vi "main.vi"(8 "error in (no error)":errorcluster) -> (0 "error out":errorcluster)   [LabVIEW 2018]
doc: "Main VI."
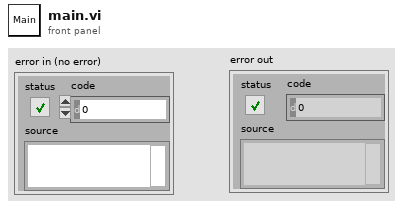
[diagram p1: front panel]
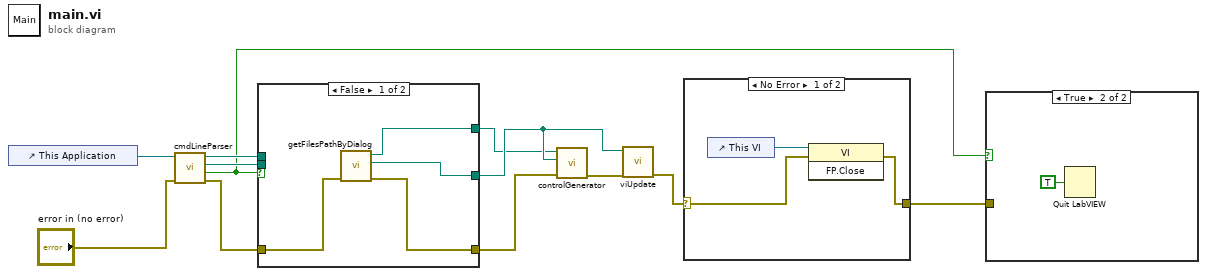
[diagram p0: block diagram]
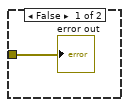
[diagram p2: hidden frame]
diagram:
  n1 = control-ref of="This Application"() -> (w3:refnum<vi>)
  n2 = call "cmdLineParser.vi"("error in (no error)"="error in (no error)", "reference"=w3) -> ("error out"=w9:errorcluster, "filesExist"=w5:bool, "pathLvlibDir"=w7:path, "pathIdl"=w8:path)  [unwired: 6 in]
  n3 = case shown="False" w5 {
    tunnel: w9 -> [w16 w19]
    tunnel: [w15 w19] -> w2
    tunnel: [w14 w18] -> w1
    tunnel: [w13 w17] -> w6
    tunnel: w8 -> [_ w18]
    tunnel: w7 -> [_ w17]
    frame False {
      n4 = call "getFilesPathByDialog.vi"("error in (no error)"=w16) -> ("error out"=w15:errorcluster, "pathLvlibDir"=w13:path, "pathIdl"=w14:path)  [unwired: 8 in]
    }
    frame True {
    }
  }
  n5 = call "controlGenerator.vi"("error in (no error)"=w2, "ControlOutputPath"=w6, "ComponentIDLFile"=w1) -> ("error out"=w11:errorcluster)  [unwired: 8 in]
  n6 = call "viUpdate.vi"("error in (no error)"=w11, "OutputPath"=w6) -> ("error out"=w12:errorcluster)  [unwired: 9 in]
  n7 = case shown="No Error" w12 {
    selector: w12 -> [w20 w23]
    tunnel: [w21 w23] -> w4
    frame No Error {
      n8 = control-ref of="This VI"() -> (w22:refnum<vi>)
      n9 = invoke class="VI" method="FP.Close"(reference=w22, error in=w20) -> (error out=w21:errorcluster)  [unwired: 1 in, 2 out]
    }
    frame Error {
    }
  }
  n10 = case shown="True" w5 {
    tunnel: w4 -> [w24 _]
    frame False {
      "error out" <- w24
    }
    frame True {
      n11 = Quit LabVIEW(quit? (T)=TRUE) -> ()
    }
  }
